vi "PID Timing Estimation.vi"(1 "Initialize?":bool, 2 "dt (s) in":dbl) -> (7 "dt (s) out":dbl)   [LabVIEW 2020, in "NI_PID_pid.lvlib"]
uses:
  <vilib>/addons/control/pid/NI_PID_pid.lvlib
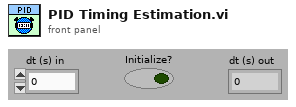
[diagram p1: front panel]
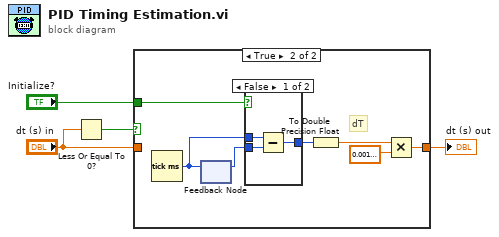
[diagram p0: block diagram]
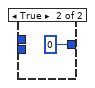
[diagram p3: hidden frame]
diagram:
  n1 = Less Or Equal To 0?(x="dt (s) in") -> (x <= 0?=w1:bool)
  n2 = case shown="True" w1 {
    tunnel: [w5 w9] -> w3
    tunnel: "dt (s) in" -> [w5 _]
    tunnel: "Initialize?" -> [_ w8]
    frame False {
    }
    frame True {
      # "dT"
      n3 = Tick Count (ms)() -> (millisecond timer value=w7:u32)
      n4 = feedback #1() -> (w6:u32)  [unwired: 1 in]
      n5 = feedback-in #1(w7) -> ()
      n6 = case shown="False" w8 {
        tunnel: [w15 u32 0] -> w11
        tunnel: w6 -> [w14 _]
        tunnel: w7 -> [w13 _]
        frame False {
          n7 = Subtract(x=w13, y=w14) -> (x-y=w15:u32)
        }
        frame True {
        }
      }
      n8 = To Double Precision Float(number=w11) -> (double precision float=w10:dbl)
      n9 = Multiply(x=w10, y=0.0010000000474974513) -> (x*y=w9:dbl)
    }
  }
  "dt (s) out" <- w3
